vi "Disabled.vi"(7 "Robot Mode":T2, 10 "Match Info":T1={"Autonomous Elapsed Seconds"=0.0, "TeleOp Elapsed Seconds"=0.0, "Disabled Elapsed Seconds"=0.0, "Visited Autonomous"=FALSE, "Visited TeleOp"=FALSE, "Visited Disabled"=FALSE, "Autonomous Settings"={"Autonomous Style"=enum."Independent", "VI Refnum"=refnum}}, 11 "Call Context":T3) -> ()   [LabVIEW 2012]
doc: "This VI is called each time a disabled packet is received from the DS. It is often used to prepare for the next robot mode, to calibrate sensors, etc."
uses:
  <vilib>/Rock Robotics/WPI/DriverStation/WPI_DriverStationDerivedRobotMode.ctl
  <vilib>/Rock Robotics/WPI/DriverStation/WPI_DriverStationRobotMode2.ctl
  <vilib>/Rock Robotics/WPI/DriverStation/WPI_DriverStationMatch Info.ctl
  Robot Global Data.vi
  <vilib>/Rock Robotics/WPI/Joystick/WPI_JoystickGetSetRefNum.vi
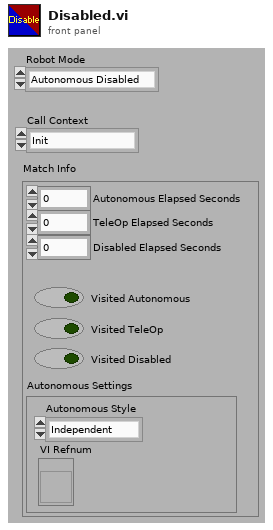
[diagram p1: front panel]
types:
  T1 = typedef "WPI_DriverStationMatch Info.ctl" = cluster{"Autonomous Elapsed Seconds":dbl, "TeleOp Elapsed Seconds":dbl, "Disabled Elapsed Seconds":dbl, "Visited Autonomous":bool, "Visited TeleOp":bool, "Visited Disabled":bool, "Autonomous Settings":cluster{"Autonomous Style":enum16{"Iterative", "Independent"}, "VI Refnum":refnum<vi>}}
  T2 = typedef "WPI_DriverStationRobotMode2.ctl" = enum16{"Autonomous Disabled", "Autonomous Enabled", "Teleop Disabled", "Teleop Enabled", "Timeout", "Finish", "Test Disabled", "Test Enabled"}
  T3 = typedef "WPI_DriverStationDerivedRobotMode.ctl" = enum16{"Init", "Execute", "Stop"}
  T4 = typedef "WPI_JoystickDevRef.ctl" = cluster{"Device":T5}
  T5 = typedef "WPI_JoystickDeviceEnum.ctl" = enum16{"USB 1", "USB 2", "USB 3", "USB 4", "Kinect 1", "Kinect 2"}
  T6 = typedef "WPI_JoystickButtonState.ctl" = cluster{"Button 1":bool, "Button 2":bool, "Button 3":bool, "Button 4":bool, "Button 5":bool, "Button 6":bool, "Button 7":bool, "Button 8":bool, "Button 9":bool, "Button 10":bool, "Button 11":bool, "Button 12":bool}
  T7 = cluster{"FlipperLeftUp":dbl, "FlipperLeftDown":dbl, "FlipperRightUp":dbl, "FlipperRightDown":dbl, "KickerLeftBack":dbl, "KickerLeftForward":dbl, "KickerRightBack":dbl, "KickerRightForward":dbl}
  T8 = typedef "WPI_MotorControlDeviceRef.ctl" = cluster{"DeviceStatus":errorcluster, "Type":enum16{"PWM", "CAN"}, "PWM":cluster{"Digital Module":T9, "PWM Channel":T10, "DeadBand":T11}, "CAN":cluster{"Device Number":u8, "Control Mode":T12, "Semaphore":T13, "Max Vout":dbl}, "Invert":bool, "TransformRef":T14, "InvTransformRef":T14}
  T9 = typedef "FPGA_TypedefDigitalModule.ctl" = enum16{"Digital Module 1", "Digital Module 2"}
  T10 = typedef "FPGA_DIOPWMChannel.ctl" = enum8{"PWM 1", "PWM 2", "PWM 3", "PWM 4", "PWM 5", "PWM 6", "PWM 7", "PWM 8", "PWM 9", "PWM 10", "Invalid"}
  T11 = typedef "WPI_PWMDeadband.ctl" = cluster{"Name":string, "maxPositivePwm":i32, "minPositivePwm":i32, "centerPwm":i32, "maxNegativePwm":i32, "minNegativePwm":i32, "angularRange":u16}
  T12 = typedef "WPI_CANJaguar_ControlMode.ctl" = enum8{"Percent VBus", "Current", "Speed", "Position", "Voltage"}
  T13 = typedef "Semaphore RefNum" = refnum<k1>
  T14 = typedef "WPI_PWMTransform_ConPane.ctl" = refnum<vi>
  T15 = typedef "WPI_ServoDeviceRef.ctl" = cluster{"DeviceStatus":errorcluster, "Digital Module":T9, "PWM Channel":T10, "DeadBand":T11}
  T16 = cluster{"Right Servo High":dbl, "Right Servo Mid":dbl, "Right Servo Low":dbl, "Left Servo High":dbl, "Left Servo Mid":dbl, "Left Servo Low":dbl}
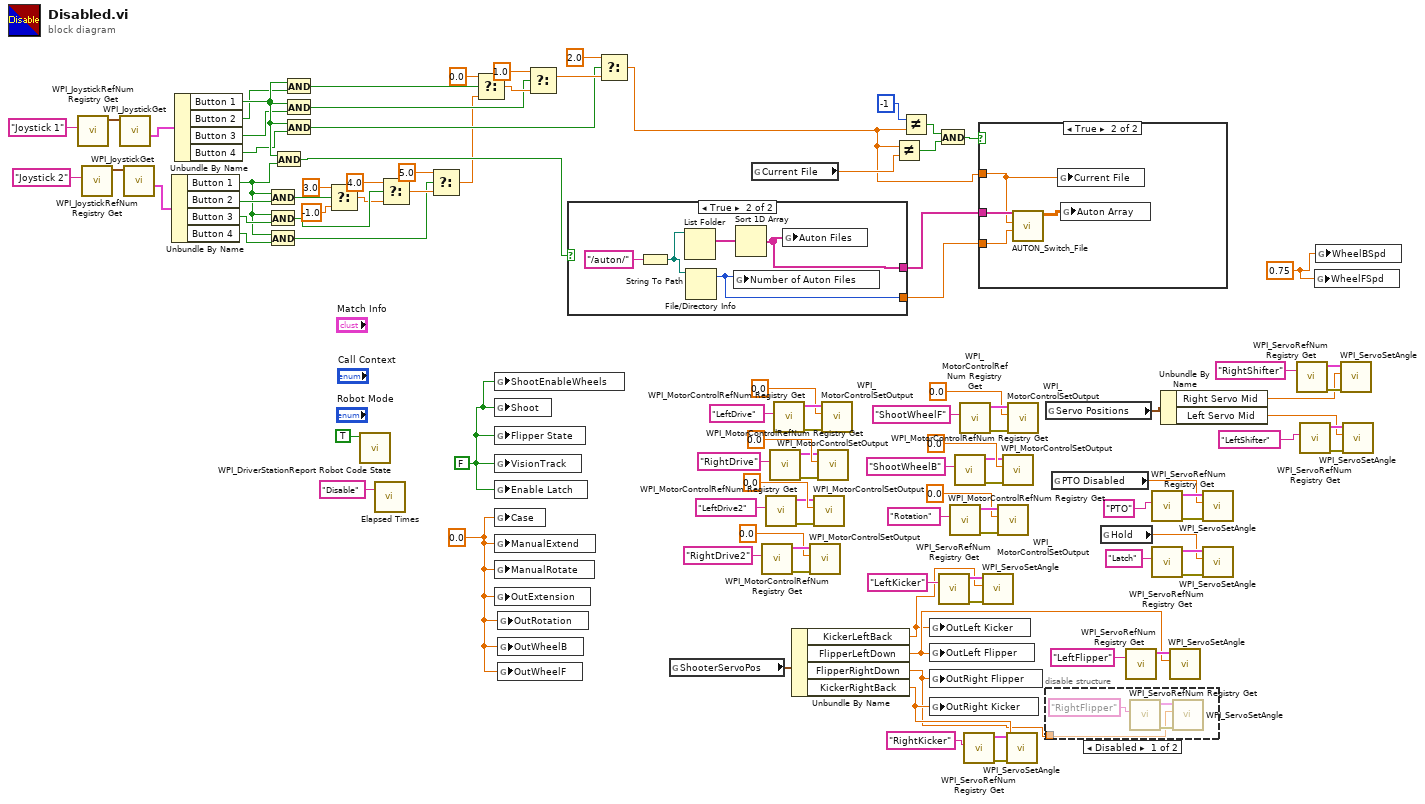
[diagram p0: block diagram]
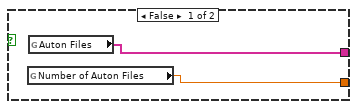
[diagram p4: hidden frame]
diagram:
  w35 = 0.75 ("Case")
  w58 = 0.0 ("Case")
  w59 = FALSE ("Enable Latch")
  n1 = call <vilib>:"WPI_JoystickRefNum Registry Get.vi"("refnum name"="Joystick 1") -> ("JoystickDevRef"=w33:T4)  [unwired: 9 in, 1 out]
  n2 = call <vilib>:"WPI_JoystickRefNum Registry Get.vi"("refnum name"="Joystick 2") -> ("JoystickDevRef"=w31:T4)  [unwired: 9 in, 1 out]
  n3 = call <vilib>:"WPI_JoystickGet.vi"("JoystickDevRef"=w33) -> ("Buttons"=w29:T6)  [unwired: 4 in, 2 out]
  n4 = call <vilib>:"WPI_JoystickGet.vi"("JoystickDevRef"=w31) -> ("Buttons"=w30:T6)  [unwired: 4 in, 2 out]
  n5 = Unbundle By Name(w30) -> ("Button 1"=w26:bool, "Button 2"=w28:bool, "Button 3"=w27:bool, "Button 4"=w25:bool)
  n6 = Unbundle By Name(w29) -> ("Button 1"=w7:bool, "Button 2"=w6:bool, "Button 3"=w5:bool, "Button 4"=w4:bool)
  n7 = And(x=w26, y=w28) -> (x .and. y?=w24:bool)
  n8 = And(x=w26, y=w27) -> (x .and. y?=w21:bool)
  n9 = And(x=w26, y=w25) -> (x .and. y?=w15:bool)
  n10 = And(x=w7, y=w26) -> (x .and. y?=w17:bool)
  n11 = And(x=w7, y=w6) -> (x .and. y?=w8:bool)
  n12 = And(x=w7, y=w5) -> (x .and. y?=w10:bool)
  n13 = And(x=w7, y=w4) -> (x .and. y?=w3:bool)
  n14 = Select(t=3.0, s=w24, f=-1.0) -> (s? t:f=w20:dbl)
  n15 = call <vilib>:"WPI_DriverStationReport Robot Code State.vi"("Disabled"=TRUE ("Autonomous")) -> ()  [unwired: 10 in, 1 out]
  n16 = call "Elapsed Times.vi"("Call Name"="Disable") -> ()  [unwired: 2 in, 1 out]
  n17 = Select(t=4.0, s=w21, f=w20) -> (s? t:f=w18:dbl)
  n18 = Select(t=5.0, s=w15, f=w18) -> (s? t:f=w2:dbl)
  n19 = Select(t=0.0, s=w8, f=w2) -> (s? t:f=w11:dbl)
  n20 = global write "Robot Global Data.vi" "ShootEnableWheels"(w59) -> ()
  n21 = global write "Robot Global Data.vi" "Shoot"(w59) -> ()
  n22 = global write "Robot Global Data.vi" "Flipper State"(w59) -> ()
  n23 = global write "Robot Global Data.vi" "VisionTrack"(w59) -> ()
  n24 = global write "Robot Global Data.vi" "Enable Latch"(w59) -> ()
  n25 = global write "Robot Global Data.vi" "Case"(w58) -> ()
  n26 = global write "Robot Global Data.vi" "ManualExtend"(w58) -> ()
  n27 = global write "Robot Global Data.vi" "ManualRotate"(w58) -> ()
  n28 = global write "Robot Global Data.vi" "OutExtension"(w58) -> ()
  n29 = global write "Robot Global Data.vi" "OutRotation"(w58) -> ()
  n30 = global write "Robot Global Data.vi" "OutWheelB"(w58) -> ()
  n31 = global write "Robot Global Data.vi" "OutWheelF"(w58) -> ()
  n32 = Select(t=1.0, s=w10, f=w11) -> (s? t:f=w13:dbl)
  n33 = case shown="True" w17 {
    tunnel: [w105 w108] -> w94
    tunnel: [w106 w107] -> w89
    frame False {
      n34 = global read "Robot Global Data.vi" "Number of Auton Files"() -> (w105:dbl)
      n35 = global read "Robot Global Data.vi" "Auton Files"() -> (w106:string[])
    }
    frame True {
      n36 = String To Path(string="/auton/") -> (path=w110:path)
      n37 = List Folder(path=w110) -> (filenames=w109:string[])  [unwired: 3 in, 3 out]
      n38 = File/Directory Info(path=w110) -> (size=w108:i64)  [unwired: 1 in, 6 out]
      n39 = global write "Robot Global Data.vi" "Number of Auton Files"(w108) -> ()
      n40 = Sort 1D Array(array=w109) -> (sorted array=w107:string[])
      n41 = global write "Robot Global Data.vi" "Auton Files"(w107) -> ()
    }
  }
  n42 = Select(t=2.0, s=w3, f=w13) -> (s? t:f=w1:dbl)
  n43 = global read "Robot Global Data.vi" "ShooterServoPos"() -> (w57:T7)
  n44 = global read "Robot Global Data.vi" "Current File"() -> (w92:dbl)
  n45 = call <vilib>:"WPI_MotorControlRefNum Registry Get.vi"("refnum name"="RightDrive2") -> ("error out"=w75:errorcluster, "MotorControlDevRef"=w74:T8)  [unwired: 9 in]
  n46 = call <vilib>:"WPI_MotorControlRefNum Registry Get.vi"("refnum name"="LeftDrive2") -> ("error out"=w68:errorcluster, "MotorControlDevRef"=w69:T8)  [unwired: 9 in]
  n47 = call <vilib>:"WPI_MotorControlRefNum Registry Get.vi"("refnum name"="RightDrive") -> ("error out"=w95:errorcluster, "MotorControlDevRef"=w96:T8)  [unwired: 9 in]
  n48 = call <vilib>:"WPI_MotorControlRefNum Registry Get.vi"("refnum name"="LeftDrive") -> ("error out"=w102:errorcluster, "MotorControlDevRef"=w101:T8)  [unwired: 9 in]
  n49 = Unbundle By Name(w57) -> ("KickerLeftBack"=w54:dbl, "FlipperLeftDown"=w55:dbl, "FlipperRightDown"=w53:dbl, "KickerRightBack"=w56:dbl)
  n50 = call <vilib>:"WPI_MotorControlSetOutput.vi"("error in (no error)"=w75, "Output"=0.0, "MotorControlDevRef"=w74) -> ()  [unwired: 6 in, 3 out]
  n51 = call <vilib>:"WPI_MotorControlSetOutput.vi"("error in (no error)"=w68, "Output"=0.0, "MotorControlDevRef"=w69) -> ()  [unwired: 6 in, 3 out]
  n52 = call <vilib>:"WPI_MotorControlSetOutput.vi"("error in (no error)"=w95, "Output"=0.0, "MotorControlDevRef"=w96) -> ()  [unwired: 6 in, 3 out]
  n53 = call <vilib>:"WPI_MotorControlSetOutput.vi"("error in (no error)"=w102, "Output"=0.0, "MotorControlDevRef"=w101) -> ()  [unwired: 6 in, 3 out]
  n54 = Not Equal?(x=w1, y=w92) -> (x != y?=w90:bool)
  n55 = Not Equal?(x=-1, y=w1) -> (x != y?=w91:bool)
  n56 = global write "Robot Global Data.vi" "OutLeft Kicker"(w54) -> ()
  n57 = global write "Robot Global Data.vi" "OutLeft Flipper"(w55) -> ()
  n58 = global write "Robot Global Data.vi" "OutRight Flipper"(w53) -> ()
  n59 = global write "Robot Global Data.vi" "OutRight Kicker"(w56) -> ()
  n60 = And(x=w91, y=w90) -> (x .and. y?=w88:bool)
  n61 = call <vilib>:"WPI_ServoRefNum Registry Get.vi"("refnum name"="LeftKicker") -> ("error out"=w60:errorcluster, "ServoDeviceRef"=w61:T15)  [unwired: 9 in]
  n62 = call <vilib>:"WPI_MotorControlRefNum Registry Get.vi"("refnum name"="Rotation") -> ("error out"=w79:errorcluster, "MotorControlDevRef"=w78:T8)  [unwired: 9 in]
  n63 = call <vilib>:"WPI_MotorControlRefNum Registry Get.vi"("refnum name"="ShootWheelB") -> ("error out"=w80:errorcluster, "MotorControlDevRef"=w81:T8)  [unwired: 9 in]
  n64 = call <vilib>:"WPI_MotorControlRefNum Registry Get.vi"("refnum name"="ShootWheelF") -> ("error out"=w87:errorcluster, "MotorControlDevRef"=w86:T8)  [unwired: 9 in]
  n65 = call <vilib>:"WPI_ServoRefNum Registry Get.vi"("refnum name"="RightKicker") -> ("error out"=w66:errorcluster, "ServoDeviceRef"=w64:T15)  [unwired: 9 in]
  n66 = case shown="True" w88 {
    tunnel: w89 -> [_ w115]
    tunnel: w94 -> [_ w114]
    tunnel: w1 -> [_ w112]
    frame False {
    }
    frame True {
      n67 = call "AUTON_Switch_File.vi"("Number of Auton Files"=w114, "Auton File"=w112, "Auton Files"=w115) -> ("Auton Array"=w113:dbl[][])  [unwired: 7 in, 1 out]
      n68 = global write "Robot Global Data.vi" "Current File"(w112) -> ()
      n69 = global write "Robot Global Data.vi" "Auton Array"(w113) -> ()
    }
  }
  n70 = call <vilib>:"WPI_ServoSetAngle.vi"("error in (no error)"=w60, "Angle"=w54, "ServoDeviceRef"=w61) -> ()  [unwired: 7 in, 2 out]
  n71 = call <vilib>:"WPI_MotorControlSetOutput.vi"("error in (no error)"=w79, "Output"=0.0, "MotorControlDevRef"=w78) -> ()  [unwired: 6 in, 3 out]
  n72 = call <vilib>:"WPI_MotorControlSetOutput.vi"("error in (no error)"=w80, "Output"=0.0, "MotorControlDevRef"=w81) -> ()  [unwired: 6 in, 3 out]
  n73 = call <vilib>:"WPI_ServoSetAngle.vi"("error in (no error)"=w66, "Angle"=w56, "ServoDeviceRef"=w64) -> ()  [unwired: 7 in, 2 out]
  n74 = call <vilib>:"WPI_MotorControlSetOutput.vi"("error in (no error)"=w87, "Output"=0.0, "MotorControlDevRef"=w86) -> ()  [unwired: 6 in, 3 out]
  n75 = global read "Robot Global Data.vi" "Servo Positions"() -> (w40:T16)
  n76 = disable-structure shown="Disabled" {
    disable-tunnel: w53 -> [w116 _]
    frame Disabled {
      n77 = call <vilib>:"WPI_ServoRefNum Registry Get.vi"("refnum name"="RightFlipper") -> ("error out"=w119:errorcluster, "ServoDeviceRef"=w117:T15)  [unwired: 9 in]
      n78 = call <vilib>:"WPI_ServoSetAngle.vi"("error in (no error)"=w119, "Angle"=w116, "ServoDeviceRef"=w117) -> ()  [unwired: 7 in, 2 out]
    }
    frame Enabled {
    }
  }
  n79 = global read "Robot Global Data.vi" "PTO Disabled"() -> (w37:dbl)
  n80 = global read "Robot Global Data.vi" "Hold"() -> (w36:dbl)
  n81 = call <vilib>:"WPI_ServoRefNum Registry Get.vi"("refnum name"="LeftFlipper") -> ("ServoDeviceRef"=w62:T15)  [unwired: 9 in, 1 out]
  n82 = call <vilib>:"WPI_ServoRefNum Registry Get.vi"("refnum name"="PTO") -> ("error out"=w43:errorcluster, "ServoDeviceRef"=w46:T15)  [unwired: 9 in]
  n83 = call <vilib>:"WPI_ServoRefNum Registry Get.vi"("refnum name"="Latch") -> ("error out"=w41:errorcluster, "ServoDeviceRef"=w42:T15)  [unwired: 9 in]
  n84 = Unbundle By Name(w40) -> ("Right Servo Mid"=w38:dbl, "Left Servo Mid"=w39:dbl)
  n85 = call <vilib>:"WPI_ServoSetAngle.vi"("Angle"=w55, "ServoDeviceRef"=w62) -> ()  [unwired: 8 in, 2 out]
  n86 = call <vilib>:"WPI_ServoSetAngle.vi"("error in (no error)"=w43, "Angle"=w37, "ServoDeviceRef"=w46) -> ()  [unwired: 7 in, 2 out]
  n87 = call <vilib>:"WPI_ServoSetAngle.vi"("error in (no error)"=w41, "Angle"=w36, "ServoDeviceRef"=w42) -> ()  [unwired: 7 in, 2 out]
  n88 = call <vilib>:"WPI_ServoRefNum Registry Get.vi"("refnum name"="RightShifter") -> ("error out"=w49:errorcluster, "ServoDeviceRef"=w50:T15)  [unwired: 9 in]
  n89 = call <vilib>:"WPI_ServoRefNum Registry Get.vi"("refnum name"="LeftShifter") -> ("error out"=w51:errorcluster, "ServoDeviceRef"=w52:T15)  [unwired: 9 in]
  n90 = global write "Robot Global Data.vi" "WheelFSpd"(w35) -> ()
  n91 = global write "Robot Global Data.vi" "WheelBSpd"(w35) -> ()
  n92 = call <vilib>:"WPI_ServoSetAngle.vi"("error in (no error)"=w49, "Angle"=w38, "ServoDeviceRef"=w50) -> ()  [unwired: 7 in, 2 out]
  n93 = call <vilib>:"WPI_ServoSetAngle.vi"("error in (no error)"=w51, "Angle"=w39, "ServoDeviceRef"=w52) -> ()  [unwired: 7 in, 2 out]
